vi "Build Full GIC.vi"(6 "Parameters":dbl[](array[numeric]), 8 "Obst Lats and Longs":cluster{"Obst Lats":dbl[], "Obst Longs":dbl[]} {"Obst Longs" format="%#_8g"; "Obst Lats" format="%#_8g"}, 9 "WP Lats and Longs":cluster{"WP Lats":dbl[], "WP Longs":dbl[]}, 10 "Num of WPs":i16, 11 "?":T3={"     Use ?\nOff       On"=[FALSE, TRUE, FALSE, TRUE], "Mode:"=FALSE, "WP Data"=0.0, "Hokuyo Port"="COM7", "Prop  Port"="COM6", "Compass Port"="", "GPS Port"=""}) -> (3 "Full GIC":T1={"     Use ?\nOff       On"=[FALSE, TRUE, FALSE, TRUE], "Mode:"=FALSE, "WP Data"=0.0, "Hokuyo Port"="COM7", "Prop  Port"="COM6", "Compass Port"="", "GPS Port"="", "Num of WPs"=0, "WP Lats and Longs"={"WP Lats"=[], "WP Longs"=[]}, "Obst Lats and Longs"={"Obst Lats"=[], "Obst Longs"=[]}, "Parameters"=[], "GPS Data"=[], "Compass"=0.0, "LMS Vector"=[], "Vision Vector"=[], "Direction Cmd"=0.0, "Speed Cmd"=0.0, "WP Vector"=[], "WP Number"=0, "Extra"=0, "SW Map"=[], "Path Cluster"={"Path x node"=[], "Path y node"=[]}} {"Obst Lats and Longs"."Obst Longs" format="%#_8g"; "Obst Lats and Longs"."Obst Lats" format="%#_8g"})   [LabVIEW 2014]
panel:
  in  "Path Cluster":T2
  in  "Extra":i16
  in  "WP Number":i32
  in  "WP Vector":dbl[](array[numeric])
  in  "Speed Cmd":dbl
  in  "Direction Cmd":dbl
  in  "GPS Data":dbl[](array[numeric])
  in  "Compass":dbl
  # "Build Full GIC"
  # "SetUp GIC Elements"
  # "Items from Top VI"
  # "Add these to GIC"
  # "Output Full GIC"
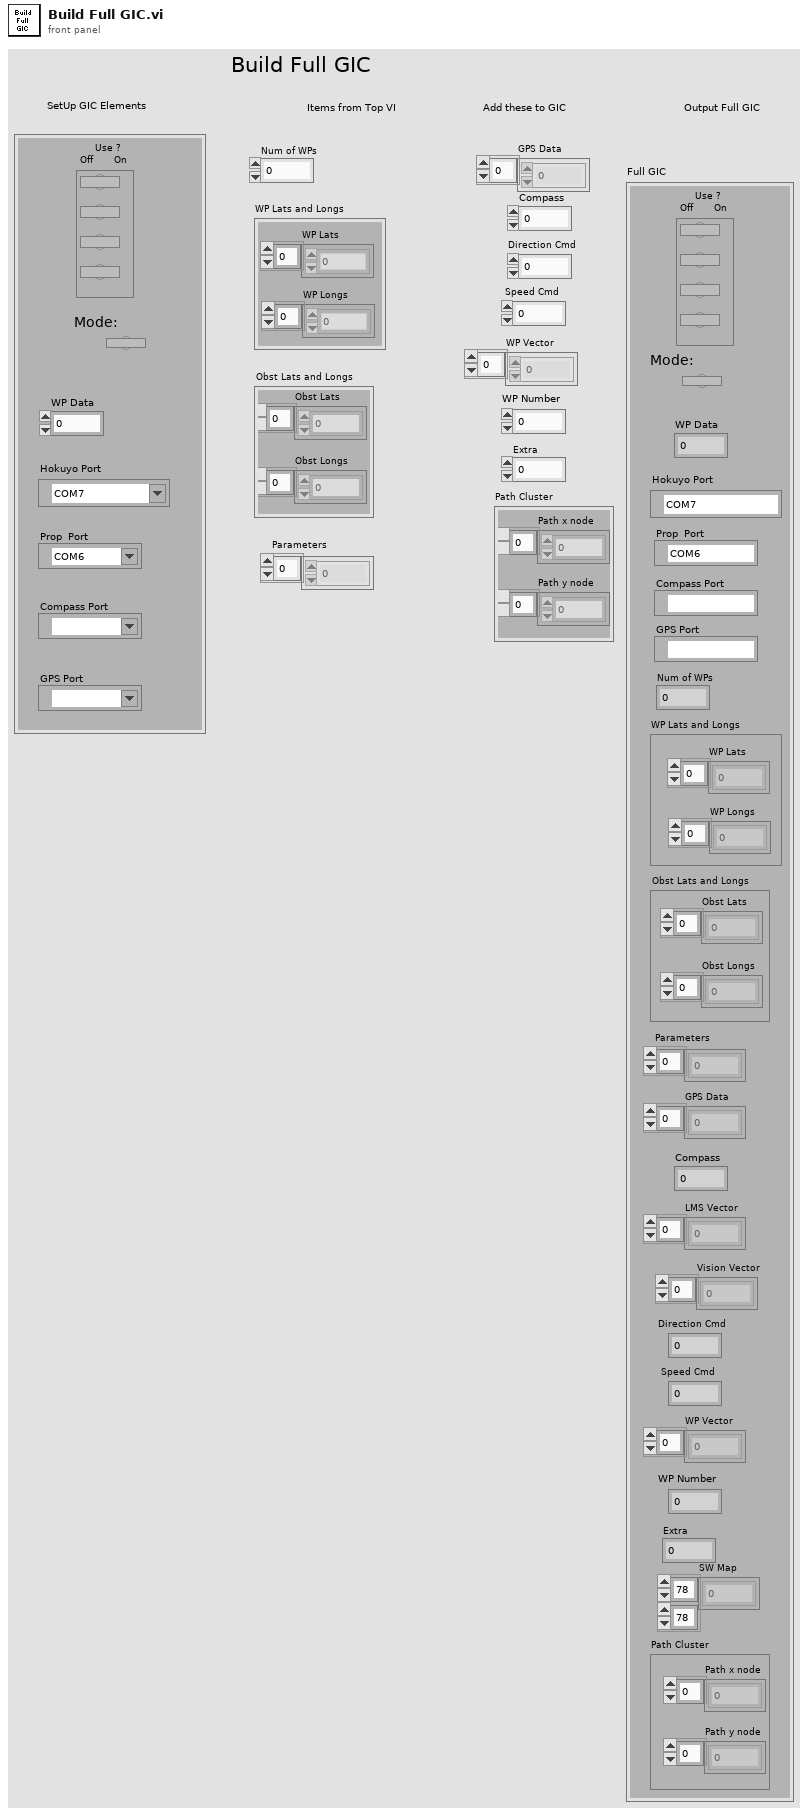
[diagram p1: front panel]
types:
  T1 = cluster{"     Use ?\nOff       On":bool[], "Mode:":bool, "WP Data":dbl, "Hokuyo Port":refnum<visa-resource-name>, "Prop  Port":refnum<visa-resource-name>, "Compass Port":refnum<visa-resource-name>, "GPS Port":refnum<visa-resource-name>, "Num of WPs":i16, "WP Lats and Longs":cluster{"WP Lats":dbl[], "WP Longs":dbl[]}, "Obst Lats and Longs":cluster{"Obst Lats":dbl[], "Obst Longs":dbl[]}, "Parameters":dbl[], "GPS Data":dbl[], "Compass":dbl, "LMS Vector":dbl[], "Vision Vector":dbl[], "Direction Cmd":dbl, "Speed Cmd":dbl, "WP Vector":dbl[], "WP Number":i32, "Extra":i16, "SW Map":i32[][], "Path Cluster":cluster{"Path x node":dbl[], "Path y node":dbl[]}}
  T2 = cluster{"Path x node":dbl[], "Path y node":dbl[]}
  T3 = cluster{"     Use ?\nOff       On":bool[], "Mode:":bool, "WP Data":dbl, "Hokuyo Port":refnum<visa-resource-name>, "Prop  Port":refnum<visa-resource-name>, "Compass Port":refnum<visa-resource-name>, "GPS Port":refnum<visa-resource-name>}
  T4 = cluster{"     Use ?\nOff       On":bool[], "Mode:":bool, "WP Data":dbl, "Hokuyo Port":refnum<visa-resource-name>, "Prop  Port":refnum<visa-resource-name>, "Compass Port":refnum<visa-resource-name>, "GPS Port":refnum<visa-resource-name>, "Num of WPs":i16, "WP Lats and Longs":cluster{"WP Lats":dbl[], "WP Longs":dbl[]}, "Obst Lats and Longs":cluster{"Obst Lats":dbl[], "Obst Longs":dbl[]}, "Parameters":dbl[], "GPS Data":dbl[], "Compass":dbl, dbl[], dbl[], "Direction Cmd":dbl, "Speed Cmd":dbl, "WP Vector":dbl[], "WP Number":i32, "Extra":i16, dbl[][], "Path Cluster":cluster{"Path x node":dbl[], "Path y node":dbl[]}}
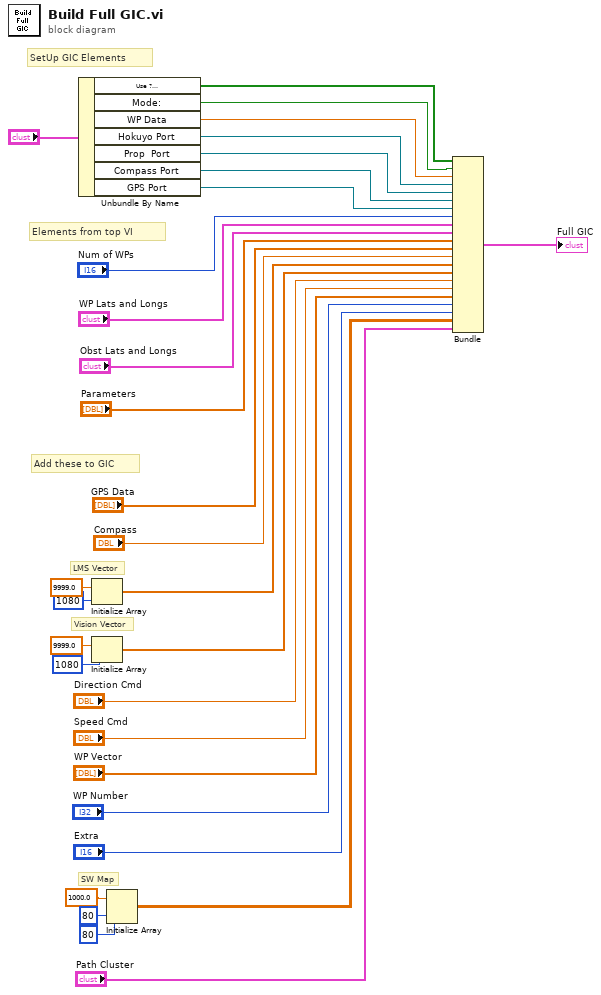
[diagram p0: block diagram]
diagram:
  # "SW Map"
  # "Vision Vector"
  # "LMS Vector"
  # "Add these to GIC"
  # "Elements from top VI"
  # "SetUp GIC Elements"
  n1 = Unbundle By Name("?") -> ("Use ?\nOff       On"=w2:bool[], "Mode:"=w3:bool, "WP Data"=w4:dbl, "Hokuyo Port"=w5:refnum<visa-resource-name>, "Prop  Port"=w23:refnum<visa-resource-name>, "Compass Port"=w22:refnum<visa-resource-name>, "GPS Port"=w21:refnum<visa-resource-name>)
  n2 = Initialize Array(9999.0 ("element"), 1080 ("dimension size")) -> (w14:dbl[])
  n3 = Initialize Array(9999.0 ("element"), 1080 ("dimension size")) -> (w13:dbl[])
  n4 = Initialize Array(1000.0 ("element"), 80 ("dimension size"), 80 ("dimension size")) -> (w7:dbl[][])
  n5 = Bundle("Use ?\nOff       On"=w2, "Mode:"=w3, "WP Data"=w4, "Hokuyo Port"=w5, "Prop  Port"=w23, "Compass Port"=w22, "GPS Port"=w21, "Num of WPs"="Num of WPs", "WP Lats and Longs"="WP Lats and Longs", "Obst Lats and Longs"="Obst Lats and Longs", "Parameters"="Parameters", "GPS Data"="GPS Data", "Compass"="Compass", w14, w13, "Direction Cmd"="Direction Cmd", "Speed Cmd"="Speed Cmd", "WP Vector"="WP Vector", "WP Number"="WP Number", "Extra"="Extra", w7, "Path Cluster"="Path Cluster") -> (→"Full GIC":T4)  [unwired: 1 in]
